vi "lj_test_top.vi"() -> ()   [LabVIEW 2025, in "LabJackEKG.lvlib"]
uses:
  LabJackEKG.lvlib
  Typedefs/LabJackData.ctl
  Typedefs/AcquisitionConfig.ctl
  StreamProducerLoopData.ctl
  <vilib>/Analysis/2dsp.llb/Real FFT.vi
  <vilib>/Analysis/NI_AALPro.lvlib
panel:
  in  "Drum Max. Accl. Factor":dbl
  out "iteration count":i32
  out "LJMScanBacklog":i32
  out "DeviceScanBacklog":i32
  in  "Display Period [ms]":i32=100
  out "fft":dbl[](graph)
  out "Waveform Graph":dbl[](graph)
  in  "LabJackConfig":T1={"Drum Reflectors"=4, "Drum Max. Samping Window [s]"=2.0, "Drum Min. Sampling Window [s]"=0.5, "Flow Max. Samping Window [s]"=1.0, "Flow Min. Sampling Window [s]"=0.25, "Pulse value [mL]"=0.0, "RMS Sampling Window [s]"=3.0, "TC Sampling Window [s]"=0.25, "TC Scale"=[1.0, 1.0], "TC Offset [V]"=[0.0, 0.0]} {"TC Offset [V]" format="%#_f"; "TC Scale" format="%#_f"; "Pulse value [mL]" format="%#_f"}
  out "Read Data":T2 {"Peak to Peak [V]" format="%#_f"; "RMS [Hz]" format="%#_f"; "CJTemp [K]" format="%#_f"; "TC [V]" format="%#_f"; "TC [degC]" format="%#_f"; "RMS [A]" format="%#_f"; "Volume [L]" format="%#_f"; "Flow [L/min]" format="%#_f"; "Spin  [RPM]" format="%#_f"}
  out "error out 2":errorcluster
  out "stop inbd":bool
  in  "error in (no error)":errorcluster
  in  "ms":u32=100
  out "error out":errorcluster={"status"=TRUE, "code"=8607, "source"="LJM_eStreamStart.vi"}
  in  "stop":bool
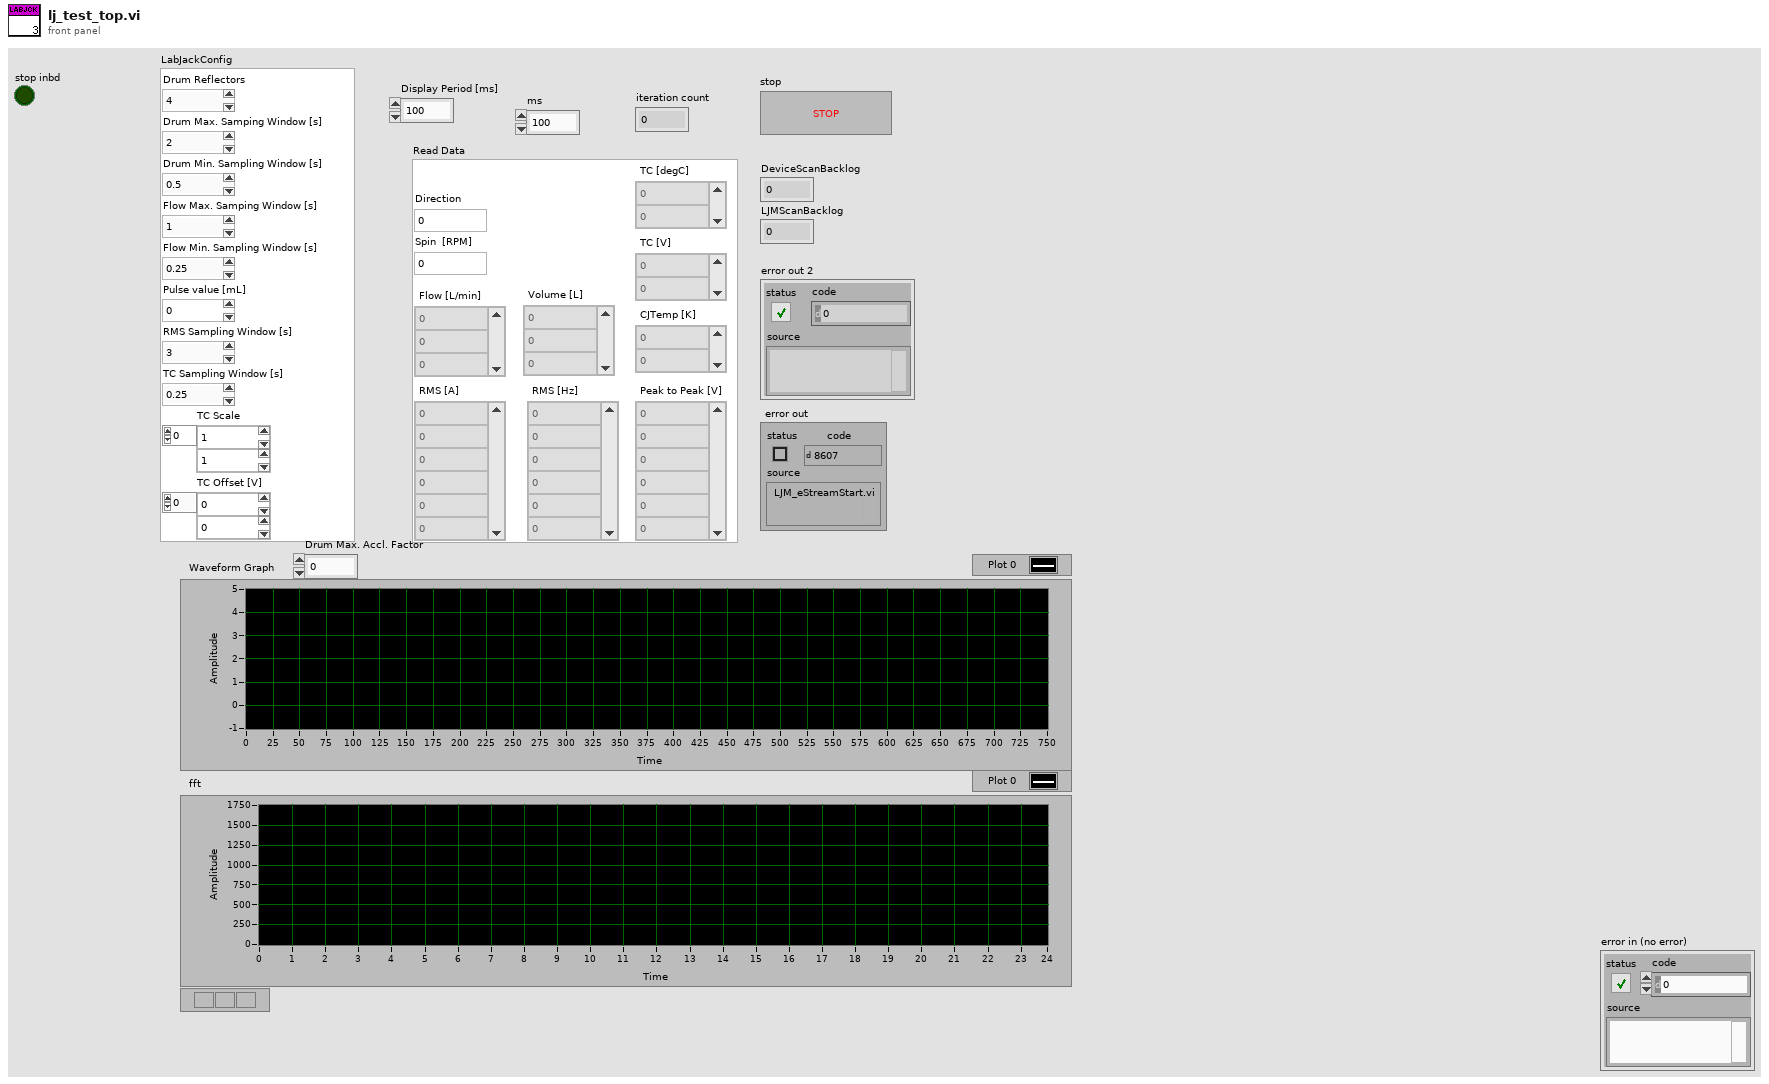
[diagram p1: front panel]
types:
  T1 = typedef "LabJackEKG.lvlib/AcquisitionConfig.ctl" = cluster{"Drum Reflectors":i64, "Drum Max. Samping Window [s]":dbl, "Drum Min. Sampling Window [s]":dbl, "Flow Max. Samping Window [s]":dbl, "Flow Min. Sampling Window [s]":dbl, "Pulse value [mL]":dbl, "RMS Sampling Window [s]":dbl, "TC Sampling Window [s]":dbl, "TC Scale":dbl[], "TC Offset [V]":dbl[]}
  T2 = typedef "LabJackEKG.lvlib/LabJackData.ctl" = cluster{"Direction":i32, "Spin  [RPM]":dbl, "Flow [L/min]":dbl[], "Volume [L]":dbl[], "RMS [A]":dbl[], "TC [degC]":dbl[], "TC [V]":dbl[], "CJTemp [K]":dbl[], "RMS [Hz]":dbl[], "Peak to Peak [V]":dbl[]}
  T3 = typedef "LabJackEKG.lvlib/StreamProducerLoopData.ctl" = cluster{"Count":i64, "Time":dbl, "Initialized":bool}
  T4 = typedef "LabJackEKG.lvlib/LabJackGlobalResources.ctl" = cluster{"DirQ":refnum<queue>, "AiQ":refnum<queue>[], "CntQ":T5[]}
  T5 = typedef "LabJackEKG.lvlib/CounterQueues.ctl" = cluster{"Events":refnum<queue>, "CurTime":refnum<queue>, "debug":refnum<queue>}
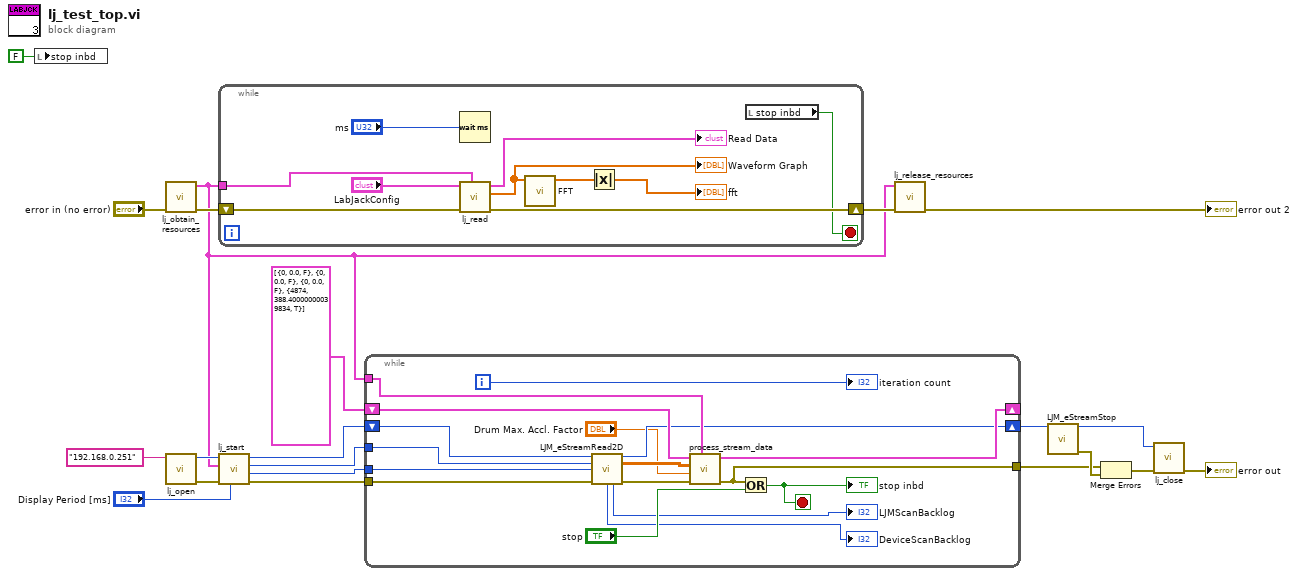
[diagram p0: block diagram]
diagram:
  n1 = local write "stop inbd"(FALSE ("stop inbd")) -> ()
  n2 = call "lj_obtain_resources.vi"("error in (no error)"="error in (no error)") -> ("error out"=w6:errorcluster, "LabJackRes"=w1:T4)  [unwired: 9 in]
  n3 = call "lj_open.vi"("IP Address (LJM_idANY )"="192.168.0.251") -> ("error out"=w21:errorcluster, "Handle"=w20:i32)  [unwired: 8 in, 1 out]
  n4 = while {
    tunnel: w1 -> [w26]
    shift-right: [w31] -> w4
    shift-left: w6 -> [w30]
    stop <- w27 stop-if-true
    n5 = Wait (ms)(milliseconds to wait="ms") -> ()  [unwired: 1 out]
    n6 = call "lj_read.vi"("Queues"=w26, "error in (no error)"=w30, "LabJackConfig"="LabJackConfig") -> ("error out"=w31:errorcluster, "subarray"=w24:dbl[], "Read Data"=→"Read Data":T2)  [unwired: 6 in]
    "Waveform Graph" <- w24
    n7 = call-poly <vilib>:"FFT.vi"("X"=w24) -> ("FFT {X}"=w23:cdb[])  [unwired: 9 in, 1 out]
    n8 = Absolute Value(x=w23) -> (abs(x)=→"fft":dbl[])
    n9 = local read "stop inbd"() -> (w27:bool)
  }
  n10 = call "lj_start.vi"("Period [ms]"="Display Period [ms]", "error in (no error)"=w21, "LabJackRes"=w1, "Handle In"=w20) -> ("error out"=w19:errorcluster, "NumReadAddresses"=w16:i32, "ScansPerRead Out"=w17:i32, "Handle Out"=w18:i32)  [unwired: 4 in]
  n11 = while {
    tunnel: w19 -> [w48]
    tunnel: [w42] -> w8
    tunnel: w17 -> [w46]
    tunnel: w16 -> [w47]
    shift-right: [w36] -> w12
    shift-left: w18 -> [w45]
    tunnel: w1 -> [w38]
    shift-right: [w40] -> _
    shift-left: T3[] [{"Count"=0, "Time"=0.0, "Initialized"=FALSE}, {"Count"=0, "Time"=0.0, "Initialized"=FALSE}, {"Count"=0, "Time"=0.0, "Initialized"=FALSE}, {"Count"=4874, "Time"=388.40000000039834, "Initialized"=TRUE}] ("Loop Data In") -> [w37]
    i -> [w33]
    stop <- w43 stop-if-true
    n12 = call <vilib>:"LJM_eStreamRead2D.vi"("Handle In"=w45, "ScansPerRead"=w46, "NumAddresses"=w47, "error in"=w48) -> ("Handle Out"=w36:i32, "aData Out"=w39:dbl[][], "DeviceScanBacklog"=→"DeviceScanBacklog":i32, "LJMScanBacklog"=→"LJMScanBacklog":i32, "error out"=w41:errorcluster)  [unwired: 7 in]
    n13 = call "process_stream_data.vi"("Queues"=w38, "error in (no error)"=w41, "Drum Max. Accl. Factor"="Drum Max. Accl. Factor", "aData Out"=w39, "Loop Data In"=w37) -> ("error out"=w42:errorcluster, "Loop Data Out"=w40:T3[])  [unwired: 5 in]
    n14 = Or(x=w42, y="stop") -> (x .or. y?=w43:bool)
    "stop inbd" <- w43
    "iteration count" <- w33
  }
  n15 = call "lj_release_resources.vi"("error in (no error)"=w4, "LabJackRes"=w1) -> ("error out"=→"error out 2":errorcluster)  [unwired: 9 in]
  n16 = call <vilib>:"LJM_eStreamStop.vi"("Handle In"=w12) -> ("Handle Out"=w11:i32, "error out"=w9:errorcluster)  [unwired: 13 in]
  n17 = Merge Errors(w8, w9) -> (w10:errorcluster)
  n18 = call "lj_close.vi"("error in"=w10, "Handle"=w11) -> ("error out"=→"error out":errorcluster)  [unwired: 9 in]
